vi "water level pid controller.vi"() -> ()   [LabVIEW 2023]
panel:
  in  "Knob":dbl(knob) scale=0.0..300.0
  out "Tank":dbl(slide) scale=0.0..10.0
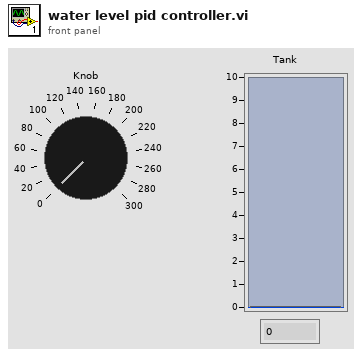
[diagram p1: front panel]
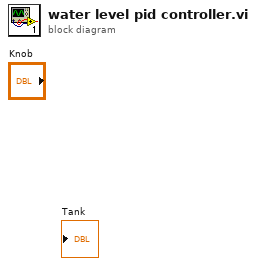
[diagram p0: block diagram]
diagram:
